vi "GAS.vi"() -> ()   [LabVIEW 2021]
uses:
  <vilib>/Instr/_visa.llb/VISA Configure Serial Port (Instr).vi
panel:
  out "NHIET DO":dbl(graph)
  out "GAS":dbl(graph)
  in  "stop":bool
  in  "VISA resource name":refnum<visa-resource-name>
  in  "TEST HE THONG":bool
  out "Den bao nhiet do":bool
  out "Den bao lua":bool
  out "Den bao gas":bool
  out "°C":dbl(knob) scale=0.0..50.0
  out "Logic 0/1":dbl(knob) scale=0.0..1.0
  out "GAS":dbl(knob) scale=0.0..1023.0
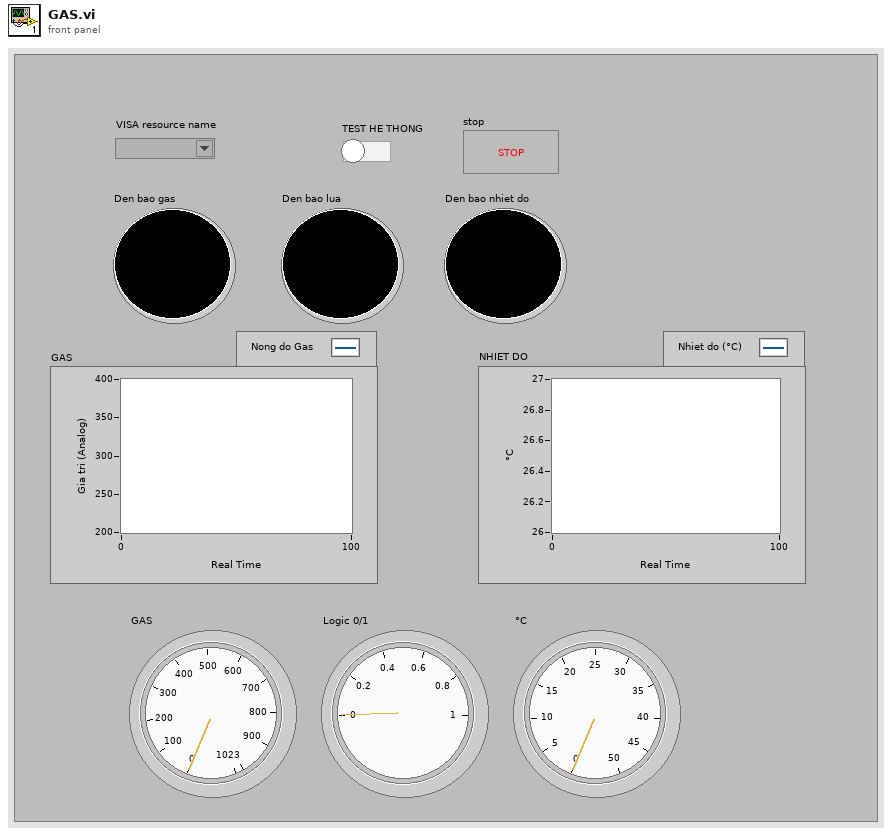
[diagram p1: front panel]
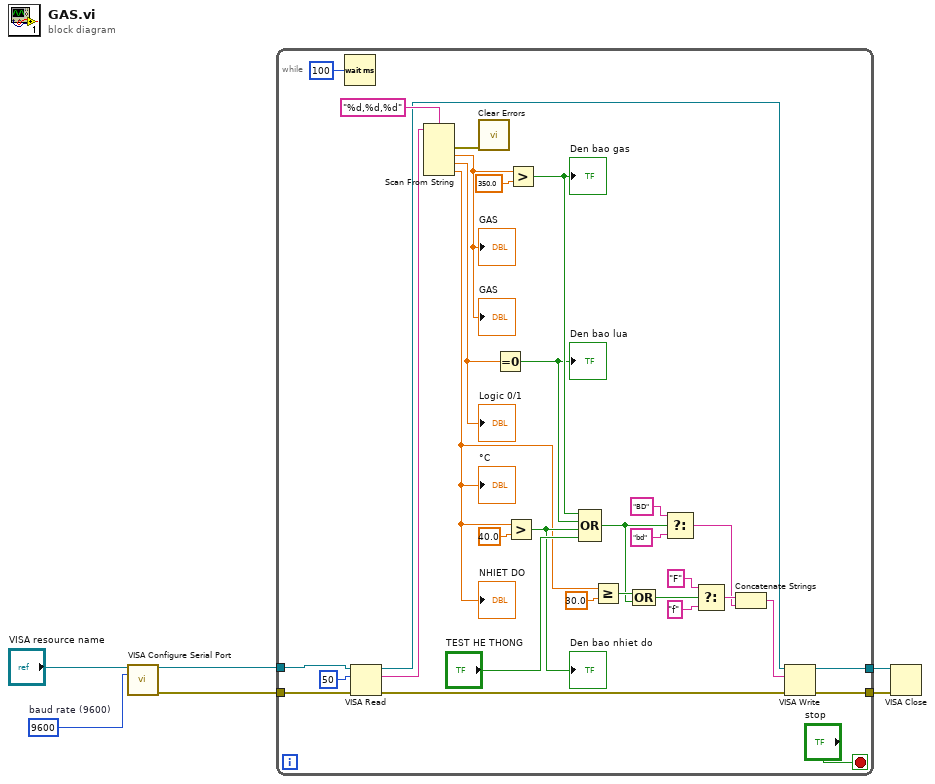
[diagram p0: block diagram]
diagram:
  w5 = u32 9600  # baud rate (9600)
  n1 = call-poly "VISA Configure Serial Port"("VISA resource name"="VISA resource name", "baud rate (9600)"=w5) -> ("VISA resource name out"=w4:refnum<visa-resource-name>, "error out"=w3:errorcluster)  [unwired: 12 in]
  n2 = while {
    tunnel: w4 -> [w36]
    tunnel: w3 -> [w35]
    tunnel: [w21] -> w2
    tunnel: [w20] -> w1
    stop <- "stop" stop-if-true
    n3 = Wait (ms)(milliseconds to wait=u32 100) -> ()  [unwired: 1 out]
    n4 = VISA Read(VISA resource name=w36, byte count=u32 50, error in (no error)=w35) -> (VISA resource name out=w22:refnum<visa-resource-name>, read buffer=w25:string, error out=w24:errorcluster)  [unwired: 1 out]
    n5 = Scan From String(format string="%d,%d,%d", input string=w25) -> (error out=w19:errorcluster, output 1=w8:dbl, output 2=w32:dbl, output 3=w7:dbl)  [unwired: 5 in, 2 out]
    "GAS" <- w8
    "Logic 0/1" <- w32
    "°C" <- w7
    "GAS" <- w8
    "NHIET DO" <- w7
    n6 = call <vilib>:"Clear Errors.vi"("error in (no error)"=w19) -> ()  [unwired: 5 in, 2 out]
    n7 = Equal To 0?(x=w32) -> (x = 0?=w14:bool)
    "Den bao lua" <- w14
    n8 = Greater?(x=w7, y=40.0) -> (0:w9:bool)
    "Den bao nhiet do" <- w9
    n9 = Greater?(x=w8, y=350.0) -> (0:w15:bool)
    "Den bao gas" <- w15
    n10 = Compound Arithmetic op=OR(w15, w14, w9, "TEST HE THONG") -> (w11:bool)
    n11 = Greater Or Equal?(x=w7, y=30.0) -> (x >= y?=w13:bool)
    n12 = Compound Arithmetic op=OR(w13, w11) -> (w12:bool)
    n13 = Select(t="BD", s=w11, f="bd") -> (s? t:f=w26:string)
    n14 = Select(t="F", s=w12, f="f") -> (s? t:f=w27:string)
    n15 = Concatenate Strings(w27, w26) -> (w23:string)
    n16 = VISA Write(VISA resource name=w22, write buffer=w23, error in (no error)=w24) -> (VISA resource name out=w21:refnum<visa-resource-name>, error out=w20:errorcluster)  [unwired: 1 out]
  }
  n17 = VISA Close(VISA resource name=w2, error in (no error)=w1) -> ()  [unwired: 1 out]
